vi "Single Trigger_fpga.vi"(4 "Continuous Trigger":bool, 5 "Stop":bool, 6 "Run":bool, 7 "Pulse params":T1, 9 "Adapter Module":enum16{"5772-DC", "5772-AC"}(ring), 10 "FPGA Card":enum16{"7976R", "7975R"}(ring), 11 "RIO Resource Name":string) -> (0 "error out":errorcluster)   [LabVIEW 2020]
uses:
  <vilib>/Utility/error.llb/Error Cluster From Error Code.vi
  <vilib>/rvi/errors/niLvFpgaAdjustHostInterfaceError.vi
  <vilib>/FPGAPlugInAG/Dynamic/niLvFpga_Close_Dynamic.vi
  <vilib>/rvi/interface/nirviReadWriteControl/nirviReadWriteControl.xnode
  Standalone FPGA/FPGA_ref.ctl
  <vilib>/rvi/interface/nirviCloseFPGA/nirviCloseFPGA.xnode
  <vilib>/rvi/interface/nirviOpenFPGA/nirviOpenFPGA.xnode
  <vilib>/FPGAPlugInAG/PXIe-7976R/niLvFpga_Open_PXIe-7976R.vi
  <vilib>/rvi/interface/common/dynamic/niFpgaDynamicAddResources.vi
  FPGA Bitfiles/aolcontrolprojec_FPGATarget_Gentrigpulse_Cnv+VIMB-cw_AC.lvbitx
  FPGA Bitfiles/aolcontrolprojec_FPGATarget2_GenTrigPulse7975_JoXGkHjNmUo.lvbitx
  NiFpgaLv.dll
  <vilib>/rvi/interface/Simulation/niFpgaSimulationCallBeginRW.vi
  FPGA Bitfiles/aolcontrolprojec_FPGATarget_GenerateTrigpuls_kZV7cFEd9rk.lvbitx
  <vilib>/FPGAPlugInAG/PXIe-7975R/niLvFpga_Open_PXIe-7975R.vi
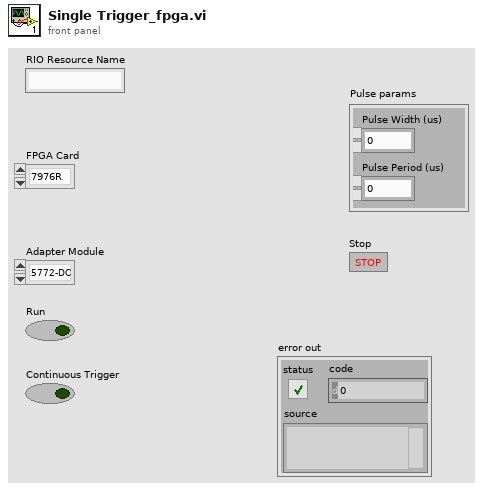
[diagram p1: front panel]
types:
  T1 = cluster{"Pulse Period (us)":u32, "Pulse Width (us)":u32}
  T2 = enum16{"Initialise FPGA ref", "Read FPGA ref", "Close FPGA Ref"}
  T3 = typedef "FPGA_ref.ctl" = refnum<k20>
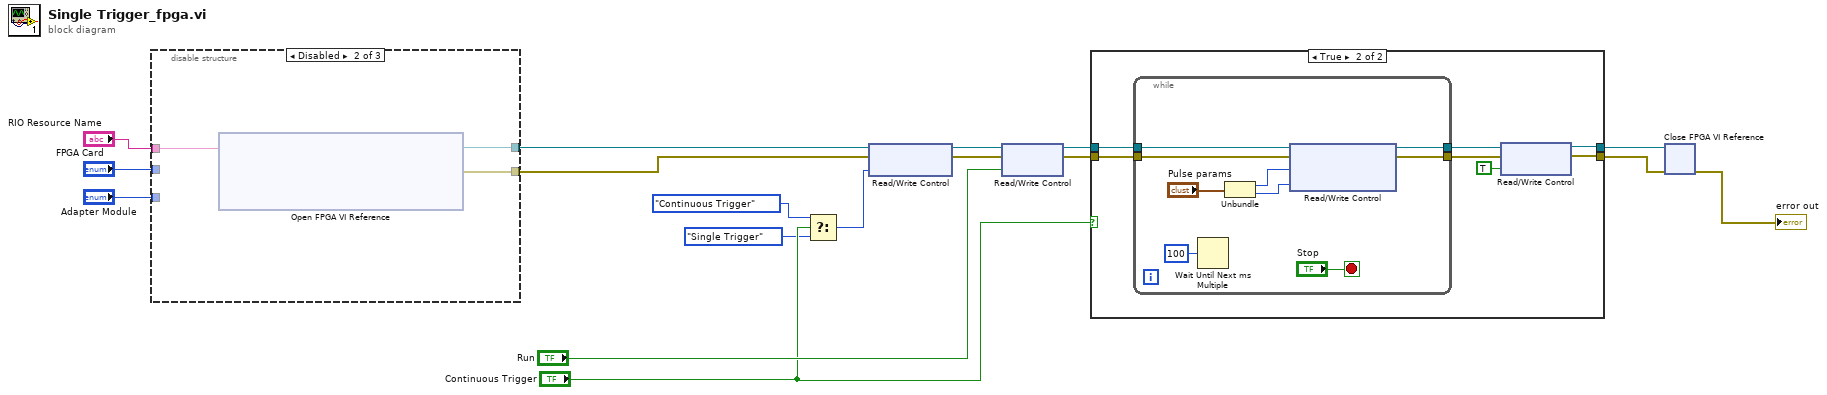
[diagram p0: block diagram]
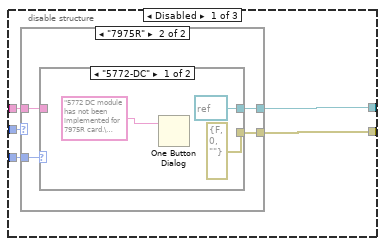
[diagram p2: hidden frame]
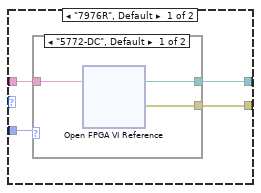
[diagram p3: hidden frame]
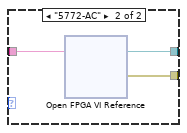
[diagram p4: hidden frame]
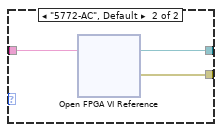
[diagram p5: hidden frame]
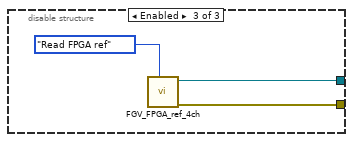
[diagram p6: hidden frame]
diagram:
  n1 = disable-structure shown="Disabled" {
    disable-tunnel: "RIO Resource Name" -> [w22 w43 _]
    disable-tunnel: "Adapter Module" -> [w21 _ _]
    disable-tunnel: "FPGA Card" -> [w20 _ _]
    disable-tunnel: [w19 w44 w46] -> w7
    disable-tunnel: [w18 w45 w47] -> w8
    frame Disabled {
      n2 = case shown="\"7975R\"" w20 {
        tunnel: [w26 w35] -> w18
        tunnel: [w25 w34] -> w19
        tunnel: w21 -> [w24 w36]
        tunnel: w22 -> [w23 w33]
        frame "7976R", Default {
          n3 = case shown="\"5772-DC\", Default" w24 {
            tunnel: [w29 w32] -> w26
            tunnel: [w28 w31] -> w25
            tunnel: w23 -> [w27 w30]
            frame "5772-DC", Default {
              n4 = xnode "Open FPGA VI Reference"("resource name"=w27) -> ("FPGA VI Reference Out"=w29:refnum<k20>, "error out"=w28:errorcluster)  [unwired: 1 in]
            }
            frame "5772-AC" {
              n5 = xnode "Open FPGA VI Reference"("resource name"=w30) -> ("FPGA VI Reference Out"=w32:refnum<k20>, "error out"=w31:errorcluster)  [unwired: 1 in]
            }
          }
        }
        frame "7975R" {
          n6 = case shown="\"5772-DC\"" w36 {
            tunnel: [refnum<k20> refnum ("FPGA VI Reference Out") w42] -> w35
            tunnel: [errorcluster {"status"=FALSE, "code"=0, "source"=""} ("error out") w41] -> w34
            tunnel: w33 -> [_ w40]
            frame "5772-DC" {
              n7 = One Button Dialog(message="5772 DC module has not been implemented for 7975R card.\nPlease check your installed hardware. ") -> ()  [unwired: 1 in, 1 out]
            }
            frame "5772-AC", Default {
              n8 = xnode "Open FPGA VI Reference"("resource name"=w40) -> ("FPGA VI Reference Out"=w42:refnum<k20>, "error out"=w41:errorcluster)  [unwired: 1 in]
            }
          }
        }
      }
    }
    frame Disabled {
      n9 = xnode "Open FPGA VI Reference"("resource name"=w43) -> ("FPGA VI Reference Out"=w45:refnum<k20>, "error out"=w44:errorcluster)  [unwired: 1 in]
    }
    frame Enabled {
      n10 = call "FGV_FPGA_ref_4ch.vi"("Action"=T2."Read FPGA ref") -> ("error out"=w46:errorcluster, "FPGA VI Reference Out"=w47:T3)  [unwired: 9 in]
    }
  }
  n11 = Select(t=enum16{"Single Trigger", "Continuous Trigger"}."Continuous Trigger" ("Trigger Type"), s="Continuous Trigger", f=enum16{"Single Trigger", "Continuous Trigger"}."Single Trigger" ("Trigger Type")) -> (s? t:f=w1:enum16{"Single Trigger", "Continuous Trigger"})
  n12 = xnode "Read/Write Control"("FPGA VI Reference In"=w8, "error in"=w7, "Trigger Type"=w1) -> ("FPGA VI Reference Out"=w6:T3, "error out"=w5:errorcluster)
  n13 = xnode "Read/Write Control"("FPGA VI Reference In"=w6, "error in"=w5, "TL Input"="Run") -> ("FPGA VI Reference Out"=w12:T3, "error out"=w11:errorcluster)
  n14 = case shown="True" "Continuous Trigger" {
    tunnel: w12 -> [w50 w57]
    tunnel: w11 -> [w49 w56]
    tunnel: [w50 w55] -> w10
    tunnel: [w49 w52] -> w9
    frame False {
    }
    frame True {
      n15 = while {
        tunnel: w57 -> [w66]
        tunnel: w56 -> [w65]
        tunnel: [w62] -> w54
        tunnel: [w61] -> w53
        stop <- "Stop" stop-if-true
        n16 = Wait Until Next ms Multiple(millisecond multiple=u32 100) -> ()  [unwired: 1 out]
        n17 = Unbundle("Pulse params") -> ("Pulse Period (us)"=w59:u32, "Pulse Width (us)"=w58:u32)
        n18 = xnode "Read/Write Control"("FPGA VI Reference In"=w66, "error in"=w65, "Pulse Period (us)"=w59, "Pulse Width (us)"=w58) -> ("FPGA VI Reference Out"=w62:T3, "error out"=w61:errorcluster)
      }
      n19 = xnode "Read/Write Control"("FPGA VI Reference In"=w54, "error in"=w53, "stop_train"=TRUE) -> ("FPGA VI Reference Out"=w55:T3, "error out"=w52:errorcluster)
    }
  }
  n20 = xnode "Close FPGA VI Reference"("FPGA VI Reference In"=w10, "error in"=w9) -> ("error out"=→"error out":errorcluster)
